vi "3C SmallRCAct.vi"   [LabVIEW 2011]
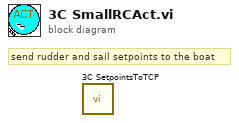
[diagram p0: block diagram]
diagram:
  # "send rudder and sail setpoints to the boat"
  n1 = call "3C SetpointsToTCP.vi"() -> ()  [unwired: 10 in, 2 out]
